vi "tm_setinputtrigger.vi"(8 "error in (no error)":errorcluster, 10 "Parameters":T1={"Mode"=1, "Polarity"=1, "Times"=1, "Delay"=0.0} {"Polarity" items=["Negative"=1, "Positive"=2]; "Mode" items=["Internal"=1, "External Edge"=2, "External Level"=4, "Software"=32, "Fast Repetition"=64, "TDI"=128, "Trigger Start"=512, "Sync Readout"=1024]}, 11 "Handle in":u32) -> (0 "error out":errorcluster, 3 "Handle out":u32)   [LabVIEW 2015]
uses:
  tmcamcon.dll
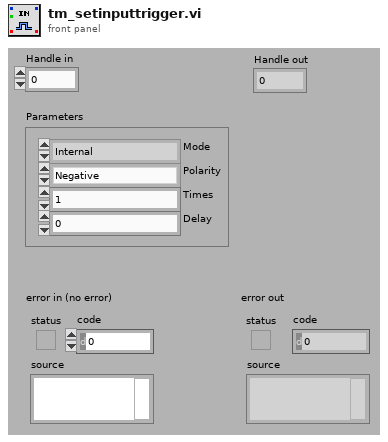
[diagram p1: front panel]
types:
  T1 = cluster{"Mode":u32, "Polarity":u32, "Times":u32, "Delay":dbl}
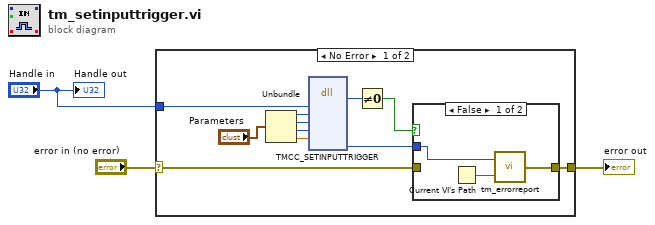
[diagram p0: block diagram]
diagram:
  n1 = case shown="No Error" "error in (no error)" {
    selector: "error in (no error)" -> [w7 w19]
    tunnel: [w4 w19] -> w2
    tunnel: "Handle in" -> [w8 _]
    frame No Error {
      n2 = Unbundle("Parameters") -> ("Mode"=w12:u32, "Polarity"=w11:u32, "Times"=w10:u32, "Delay"=w9:dbl)
      n3 = dll-call lib="tmcamcon.dll" fn="TMCC_SETINPUTTRIGGER"("HDCAM"=w8, "mode"=w12, "polarity"=w11, "times"=w10, "delay"=w9) -> ("return type"=w14:u32, "Erval"=w6:i32)  [unwired: 9 in, 2 out]
      n4 = Not Equal To 0?(x=w14) -> (x != 0?=w5:bool)
      n5 = case shown="False" w5 {
        tunnel: w7 -> [_ w18]
        tunnel: [w16 w18] -> w4
        tunnel: w6 -> [w15 _]
        frame False {
          n6 = Current VI's Path() -> (path=w17:path)
          n7 = call "tm_errorreport.vi"("Source"=w17, "Error"=w15) -> ("error out"=w16:errorcluster)
        }
        frame True {
        }
      }
    }
    frame Error {
    }
  }
  "error out" <- w2
  "Handle out" <- "Handle in"
